vi "HTML Report Alignment Tag Attribute.vi"(5 "align (default)":T1, 6 "name (ALIGN)":string="ALIGN", 7 "tag attributes in":string) -> (3 "tag attributes out":string)   [LabVIEW 2017, in "NI_ReportGenerationCore.lvlib"]
doc: "Constructs the horizontal ALIGN attribute."
uses:
  <vilib>/Utility/NIReport.llb/NI_ReportGenerationCore.lvlib
  <vilib>/Utility/NIReport.llb/HTML Report Text Alignment.ctl
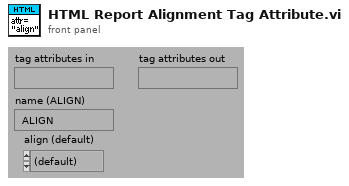
[diagram p1: front panel]
types:
  T1 = typedef "NI_ReportGenerationCore.lvlib/HTML Report Text Alignment.ctl" = enum16{"(default)", "LEFT", "CENTER", "RIGHT"}
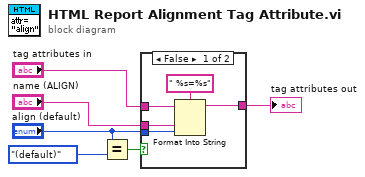
[diagram p0: block diagram]
diagram:
  n1 = Equal?(x="align (default)", y=enum16{"(default)", "LEFT", "CENTER", "RIGHT"}."(default)") -> (x = y?=w5:bool)
  n2 = case shown="False" w5 {
    tunnel: [w10 w12] -> w3
    tunnel: "align (default)" -> [w8 _]
    tunnel: "tag attributes in" -> [w9 w12]
    tunnel: "name (ALIGN)" -> [w7 _]
    frame False {
      n3 = Format Into String(format string=" %s=%s", initial string=w9, w7, w8) -> (resulting string=w10:string)  [unwired: 1 in, 1 out]
    }
    frame True {
    }
  }
  "tag attributes out" <- w3
